vi "Simulator.vi"() -> ()   [LabVIEW 2023]
panel:
  in  "Outputs":cluster{"Cooled Coolant (mB/t)":i64}
  out "Temperature (K)":dbl
  out "Heating Rate (mB/t)":i64
  in  "Fuel Input (mB/t)":i64
  in  "Coolant Type":enum16{"Water", "Sodium"}(ring)
  in  "Activate":bool
  in  "Height (m)":i32=4 min=4 max=18 step=1
  in  "Width (m)":i32=3 min=3 max=18 step=1
  in  "Length (m)":i32=3 min=3 max=18 step=1
  in  "Burn Rate (mB/t)":dbl min=0.0 max=615.0
  in  "stop":bool
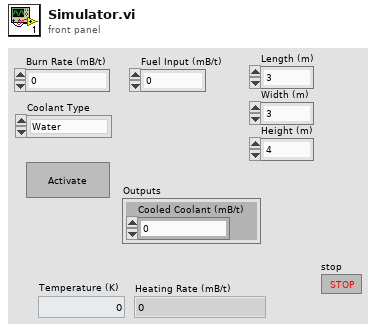
[diagram p1: front panel]
types:
  T1 = typedef "Reactor Build Properties.ctl" = cluster{"Fuel Rods":i32, "Control Rods":i32, "Volume (m³)":i32, "Fuel Surface Area (m²)":i32, "Cooled Coolant Tank (mB)":i32, "Fuel Capacity (mB)":i64, "Heat Capacity (J/K)":dbl, "Max Burn Rate":i64, "Max Heating Rate (mB/t)":i64, "Boil Efficiency":dbl, "Coolant Type":enum16{"Water", "Sodium"}, "Heated Coolant Tank (mB)":i64}
  T2 = cluster{"Waste (mB/t)":i64, "Heated Coolant (mB/t)":i64}
  T3 = typedef "Turbine Build Properties.ctl" = cluster{"Volume (m³)":i32, "Rotor Height (m)":i32, "Condensers":i32, "Vents":i32, "Rotor Blades":i32, "Coils":i32, "Dispersers":i32, "Steam Tank (mB)":i64, "Energy Capacity (FE)":ext, "Vent Flow Rate (mB/t)":dbl, "Max Water Return (mB/t)":i32, "Area (m²)":i32, "Inner Area (m²)":i32}
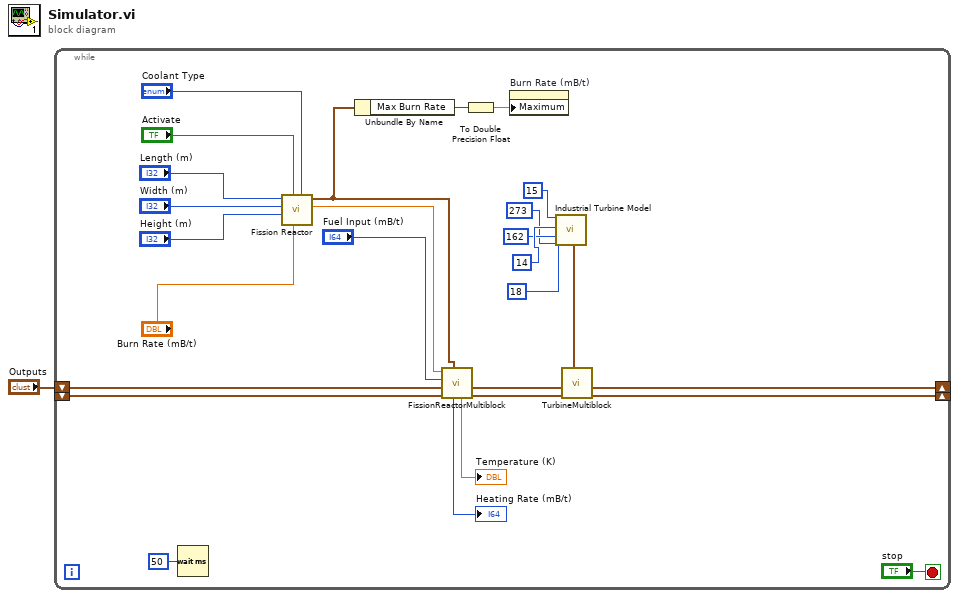
[diagram p0: block diagram]
diagram:
  n1 = while {
    shift-right: [w9] -> _
    shift-left: _ -> [w14]
    shift-right: [w8] -> _
    shift-left: "Outputs" -> [w12]
    stop <- "stop" stop-if-true
    n2 = Wait (ms)(milliseconds to wait=u32 50) -> ()  [unwired: 1 out]
    n3 = call "Fission Reactor.vi"("Coolant Type"="Coolant Type", "Burn Rate (mB/t)"="Burn Rate (mB/t)", "Activate"="Activate", "Height (m)"="Height (m)", "Width (m)"="Width (m)", "Length (m)"="Length (m)") -> ("Actual Burn Rate (mB/t)"=w15:dbl, "Computed Build Properties"=w16:T1)  [unwired: 2 in, 2 out]
    n4 = Unbundle By Name(w16) -> ("Max Burn Rate"=w20:i64)
    n5 = call "FissionReactorMultiblock.vi"("Reactor Build Properties"=w16, "Output Rejection"=w14, "Inputs"=w12, "Fuel Input (mB/t)"="Fuel Input (mB/t)", "Burn Rate (mB/t)"=w15) -> ("Input Rejection"=w10:cluster{"Cooled Coolant (mB/t)":i64}, "Outputs"=w11:T2, "Temperature (K)"=→"Temperature (K)":dbl, "Heating Rate (mB/t)"=→"Heating Rate (mB/t)":i64)  [unwired: 3 in]
    n6 = To Double Precision Float(number=w20) -> (double precision float=w19:dbl)
    n7 = property on="Burn Rate (mB/t)" class="DigNum (strict)"("Maximum"=w19) -> ()  [unwired: 2 in, 2 out]
    n8 = call "Industrial Turbine Model.vi"("Width (m)"=15, "Height (m)"=18, "Rotor Height"=14, "Condensers"=162, "Vents"=273) -> ("Turbine Build Properties"=w7:T3)  [unwired: 6 in, 8 out]
    n9 = call "TurbineMultiblock.vi"("Turbine Build Properties"=w7, "Output Rejection"=w10, "Inputs"=w11) -> ("Input Rejection"=w9:T2, "Outputs"=w8:cluster{"Cooled Coolant (mB/t)":i64})  [unwired: 7 in]
  }
